vi "DP-Add to comparison list.vi"(0 "Comparison list":T1, 5 "Data folder ref":refnum<vi>, 7 "File listbox ref":refnum<vi>) -> (4 "Comparison list out":T1)   [LabVIEW 2020]
uses:
  Typedefs/DP-Comparison List.ctl
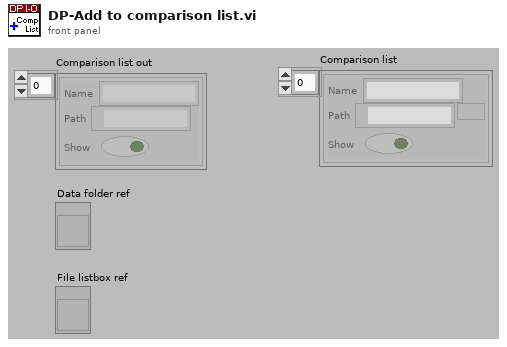
[diagram p1: front panel]
types:
  T1 = typedef "DP-Comparison List.ctl" = cluster{"Name":string, "Path":path, "Show":bool}[]
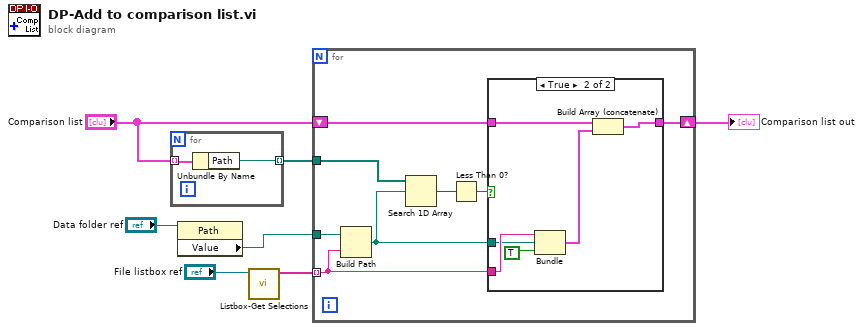
[diagram p0: block diagram]
diagram:
  n1 = for {
    tunnel: "Comparison list" -> [w9] mode=indexing
    tunnel: [w8] -> w5 mode=indexing
    n2 = Unbundle By Name(w9) -> ("Path"=w8:path)
  }
  n3 = property class="Path"(reference="Data folder ref") -> ("Value"=w3:path)  [unwired: 1 in, 2 out]
  n4 = call "Listbox-Get Selections.vi"("Listbox Ref"="File listbox ref") -> ("Selections"=w4:string[])  [unwired: 9 in, 1 out]
  n5 = for {
    tunnel: w3 -> [w17]
    tunnel: w4 -> [w10] mode=indexing
    tunnel: w5 -> [w16]
    shift-right: [w12] -> w7
    shift-left: "Comparison list" -> [w13]
    n6 = Build Path(base path=w17, name or relative path=w10) -> (appended path=w11:path)
    n7 = Search 1D Array(1D array=w16, element=w11) -> (index of element=w15:i32)  [unwired: 1 in]
    n8 = Less Than 0?(x=w15) -> (x < 0?=w14:bool)
    n9 = case shown="True" w14 {
      tunnel: [w18 w23] -> w12
      tunnel: w13 -> [w18 w24]
      tunnel: w11 -> [_ w21]
      tunnel: w10 -> [_ w22]
      frame False {
      }
      frame True {
        n10 = Bundle(w22, "appended path"=w21, TRUE) -> (w19:cluster{string, "appended path":path, bool})  [unwired: 1 in]
        n11 = Build Array (concatenate)(w24, w19) -> (w23:T1)
      }
    }
  }
  "Comparison list out" <- w7
